vi "XYMovingPart_WangYunong.vi"() -> ()   [LabVIEW 2013]
uses:
  <vilib>/Instr/_visa.llb/VISA Configure Serial Port (Instr).vi
panel:
  in  "Mov speed(mm/s)":dbl format="%#_13g"
  in  "Y pole":refnum<visa-resource-name>
  in  "X pole":refnum<visa-resource-name>
  out "XY Graph":cluster{dbl[], dbl[]}(graph)
  out "Time":dbl
  out "y step":dbl
  out "x step":dbl
  out "Case":i16
  out "Y":i32
  out "X":i32
  out "Chosen Point":dbl[][](array[numeric])
  in  "Size input solution":enum16{"Dynamic Size", "Fixed Size"}(ring)=enum."Fixed Size"
  in  "Polygon Point":dbl[][](array[numeric])
  in  "Y move Maximum / mm":dbl
  in  "X move Maximum / mm":dbl
  in  "Y step / mm":dbl
  in  "X step / mm":dbl
  in  "Initial YPos / mm":dbl
  in  "Initial XPos / mm":dbl
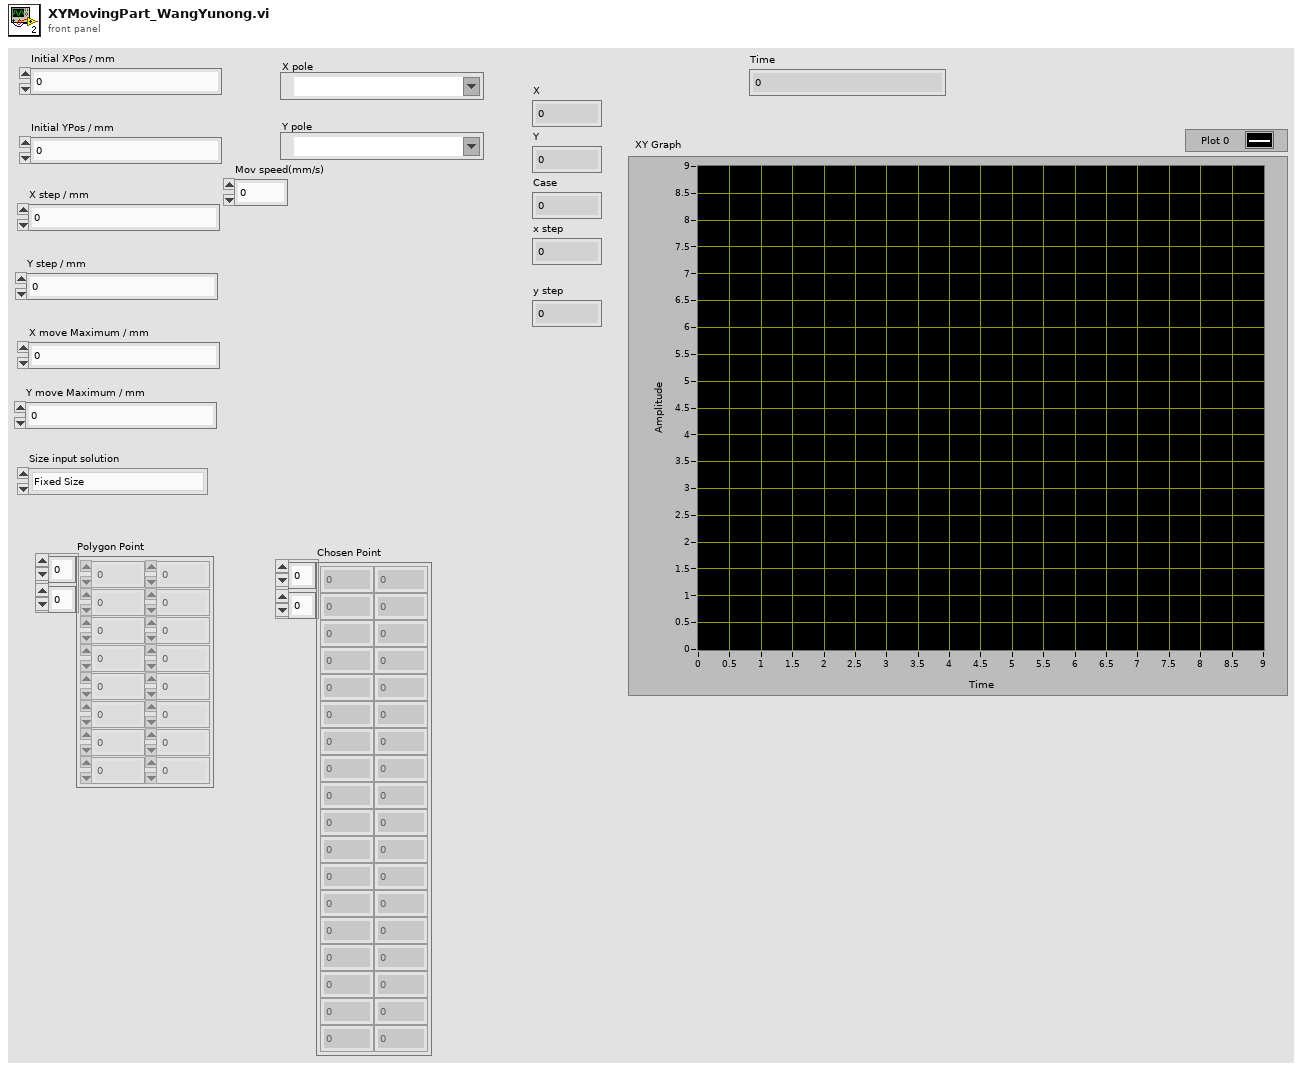
[diagram p1: front panel]
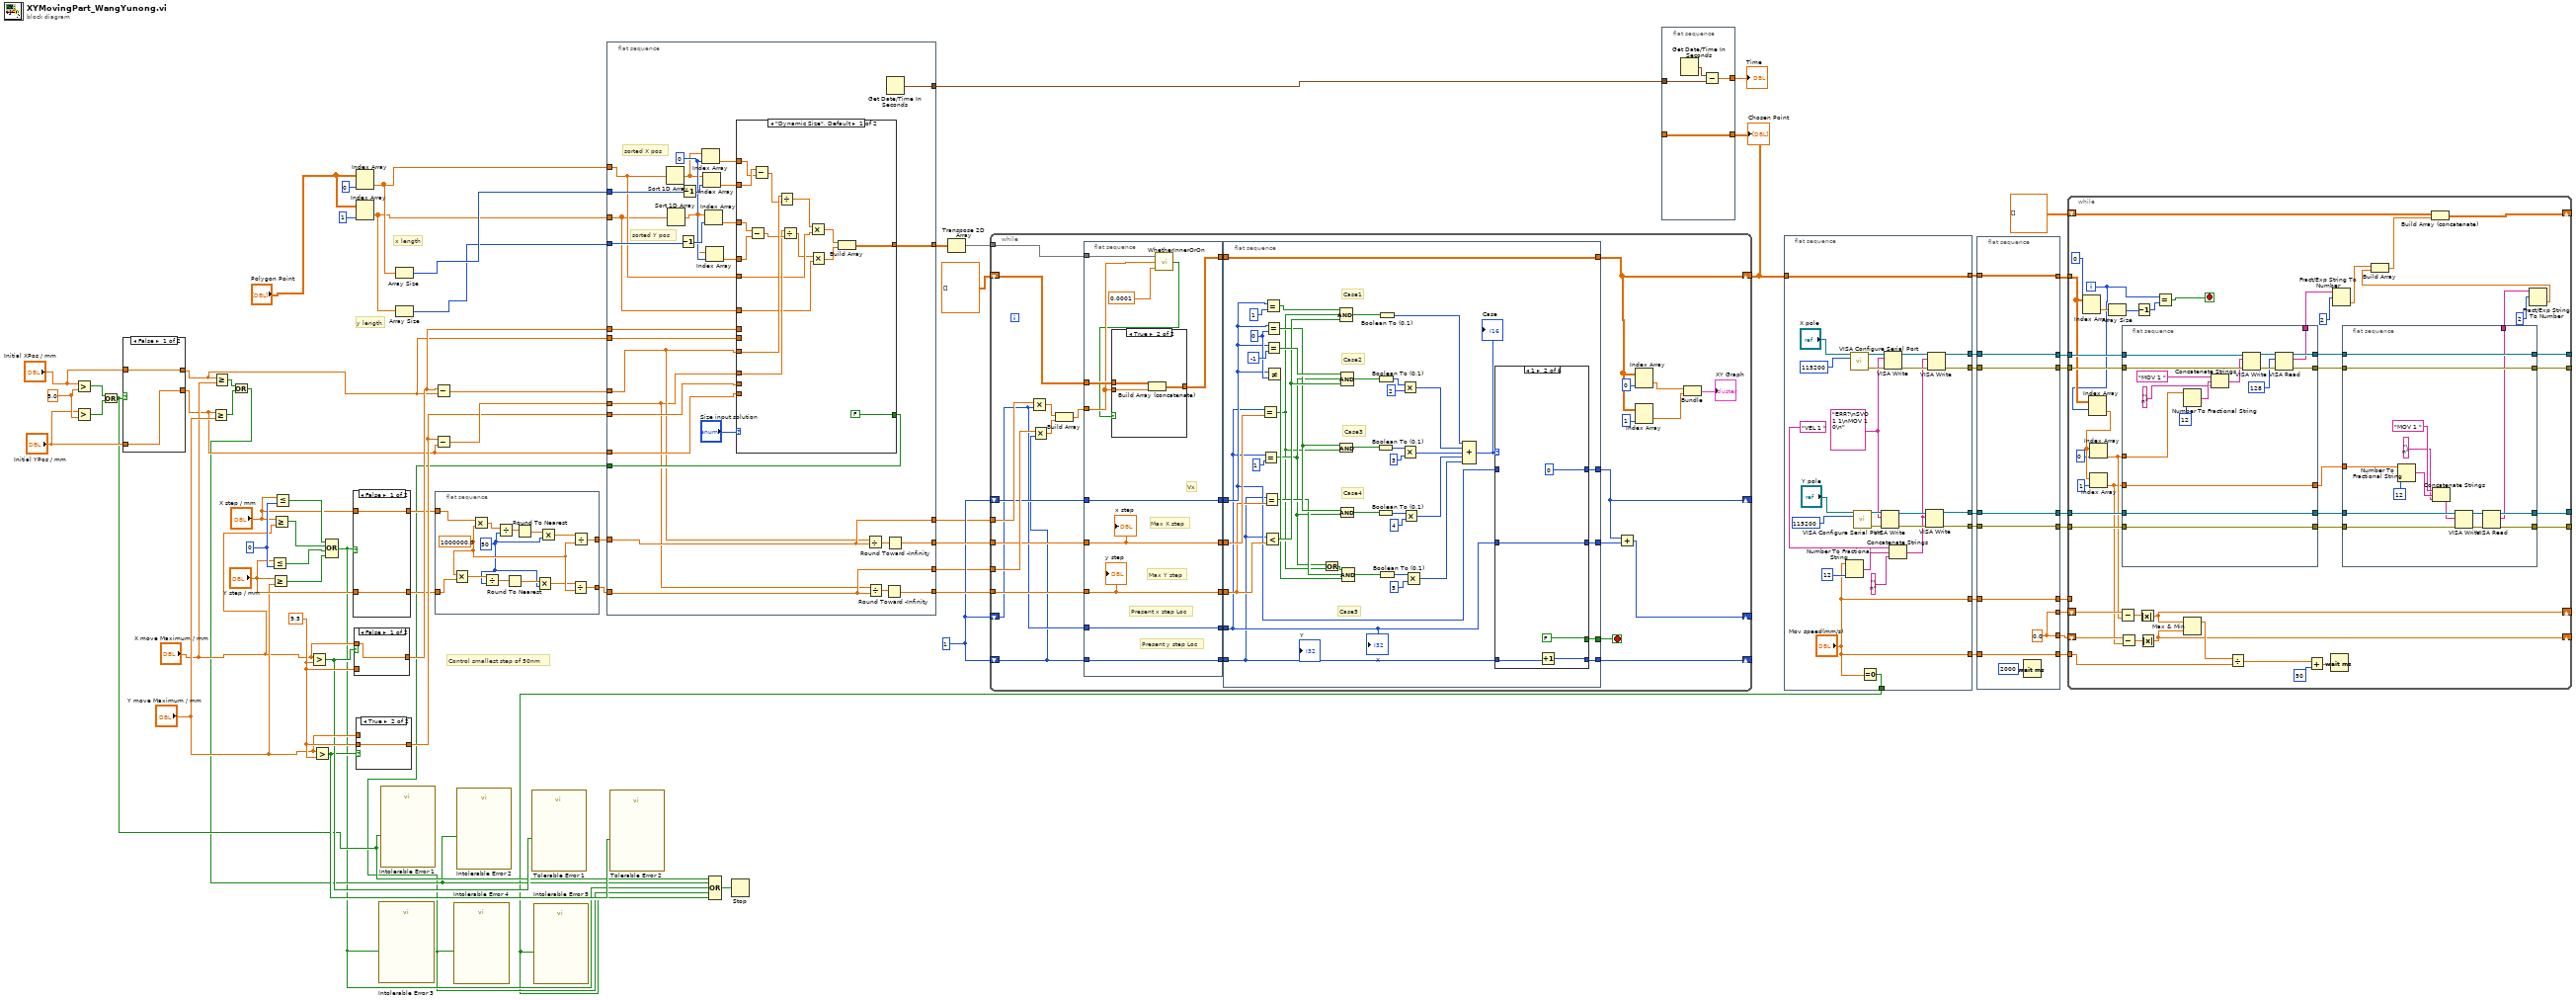
[diagram p0: block diagram]
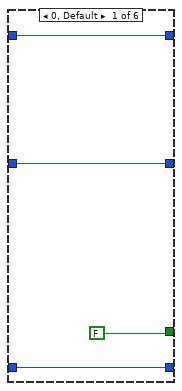
[diagram p2: hidden frame]
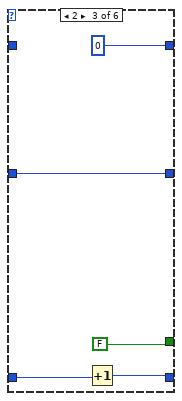
[diagram p3: hidden frame]
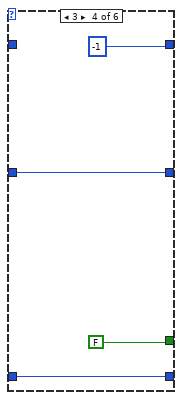
[diagram p4: hidden frame]
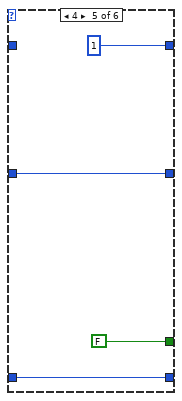
[diagram p5: hidden frame]
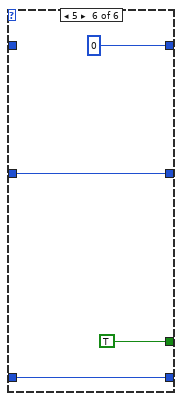
[diagram p6: hidden frame]
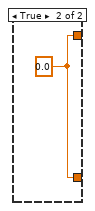
[diagram p8: hidden frame]
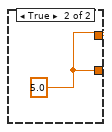
[diagram p11: hidden frame]
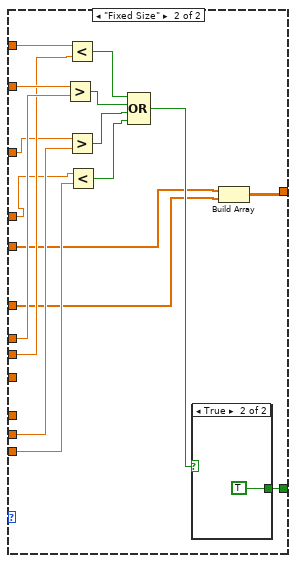
[diagram p12: hidden frame]
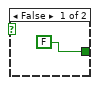
[diagram p13: hidden frame]
diagram:
  w33 = 1
  w65 = 0
  w66 = 9.5
  w71 = 5.0
  # "Control smallest step of 50nm"
  # "y length"
  # "x length"
  n1 = Greater?(x="Initial XPos / mm", y=w71) -> (0:w70:bool)
  n2 = Greater?(x="Initial YPos / mm", y=w71) -> (0:w69:bool)
  n3 = Or(x=w70, y=w69) -> (x .or. y?=w8:bool)
  n4 = case shown="False" w8 {
    tunnel: "Initial XPos / mm" -> [w73 _]
    tunnel: "Initial YPos / mm" -> [w72 _]
    tunnel: [w73 w74] -> w42
    tunnel: [w72 w74] -> w40
    frame False {
    }
    frame True {
      w74 = 5.0
    }
  }
  n5 = Greater Or Equal?(x=w40, y="Y move Maximum / mm") -> (x >= y?=w48:bool)
  n6 = Greater Or Equal?(x=w42, y="X move Maximum / mm") -> (x >= y?=w49:bool)
  n7 = Or(x=w49, y=w48) -> (x .or. y?=w7:bool)
  n8 = Less Or Equal?(x="Y step / mm", y=w65) -> (x <= y?=w62:bool)
  n9 = Greater Or Equal?(x="Y step / mm", y="Y move Maximum / mm") -> (x >= y?=w61:bool)
  n10 = Greater Or Equal?(x="X step / mm", y="X move Maximum / mm") -> (x >= y?=w63:bool)
  n11 = Less Or Equal?(x="X step / mm", y=w65) -> (x <= y?=w64:bool)
  n12 = Greater?(x="X move Maximum / mm", y=w66) -> (0:w45:bool)
  n13 = Greater?(x="Y move Maximum / mm", y=w66) -> (0:w44:bool)
  n14 = Compound Arithmetic op=OR(w64, w63, w62, w61) -> (w6:bool)
  n15 = case shown="False" w6 {
    tunnel: "X step / mm" -> [w76 _]
    tunnel: "Y step / mm" -> [w75 _]
    tunnel: [w76 w77] -> w39
    tunnel: [w75 w77] -> w38
    frame False {
    }
    frame True {
      w77 = 0.0
    }
  }
  n16 = case shown="False" w45 {
    tunnel: w66 -> [_ w79]
    tunnel: "X move Maximum / mm" -> [w78 _]
    tunnel: [w78 w79] -> w43
    frame False {
    }
    frame True {
    }
  }
  n17 = Index Array(array="Polygon Point", index (col)=1 ("disabled index (col)")) -> (element=w54:dbl[])  [unwired: 1 in]
  n18 = case shown="True" w44 {
    tunnel: w66 -> [_ w81]
    tunnel: "Y move Maximum / mm" -> [w80 _]
    tunnel: [w80 w81] -> w41
    frame False {
    }
    frame True {
    }
  }
  n19 = Index Array(array="Polygon Point", index (col)=0 ("disabled index (col)")) -> (element=w56:dbl[])  [unwired: 1 in]
  n20 = call "Intolerable Error 3"("Enable"=w6) -> ()  [unwired: 9 in, 2 out]
  n21 = call "Intolerable Error 1"("Enable"=w8) -> ()  [unwired: 9 in, 2 out]
  n22 = Array Size(array=w56) -> (size(s)=w55:i32)
  n23 = Array Size(array=w54) -> (size(s)=w53:i32)
  n24 = Subtract(x=w43, y=w42) -> (x-y=w47:dbl)
  n25 = Subtract(x=w41, y=w40) -> (x-y=w46:dbl)
  n26 = flat-sequence {
    tunnel: w39 -> [w95]
    tunnel: w38 -> [w92]
    tunnel: [w88] -> w37
    tunnel: [w87] -> w36
    frame #0 {
      w84 = 50
      w89 = 1000000.0
      n27 = Multiply(x=w89, y=w92) -> (x*y=w91:dbl)
      n28 = Multiply(x=w95, y=w89) -> (x*y=w94:dbl)
      n29 = Divide(x=w91, y=w84) -> (x/y=w90:dbl)
      n30 = Divide(x=w94, y=w84) -> (x/y=w93:dbl)
      n31 = Round To Nearest(number=w90) -> (nearest integer value=w85:dbl)
      n32 = Round To Nearest(number=w93) -> (nearest integer value=w86:dbl)
      n33 = Multiply(x=w85, y=w84) -> (x*y=w83:dbl)
      n34 = Multiply(x=w86, y=w84) -> (x*y=w82:dbl)
      n35 = Divide(x=w83, y=w89) -> (x/y=w87:dbl)
      n36 = Divide(x=w82, y=w89) -> (x/y=w88:dbl)
    }
  }
  n37 = call "Intolerable Error 4"("Enable"=w5) -> ()  [unwired: 9 in, 2 out]
  n38 = call "Intolerable Error 2"("Enable"=w7) -> ()  [unwired: 9 in, 2 out]
  n39 = call "Tolerable Error 1"("Enable"=w45) -> ()  [unwired: 9 in, 2 out]
  n40 = call "Intolerable Error 5"("Enable"=w4) -> ()  [unwired: 9 in, 2 out]
  n41 = flat-sequence {
    tunnel: w55 -> [w123]
    tunnel: w53 -> [w121]
    tunnel: w56 -> [w116]
    tunnel: w54 -> [w115]
    tunnel: w47 -> [w99]
    tunnel: w46 -> [w97]
    tunnel: w43 -> [w110]
    tunnel: w42 -> [w109]
    tunnel: w41 -> [w108]
    tunnel: w40 -> [w107]
    tunnel: [w106] -> w5
    tunnel: w37 -> [w100]
    tunnel: w36 -> [w98]
    tunnel: [w105] -> w29
    tunnel: [w102] -> w35
    tunnel: [w101] -> w34
    tunnel: [w98] -> w32
    tunnel: [w100] -> w31
    tunnel: [w96] -> w27
    frame #0 {
      w119 = 0 ("index")
      # "sorted Y pos"
      # "sorted X pos"
      n42 = Sort 1D Array(array=w116) -> (sorted array=w117:dbl[])
      n43 = Sort 1D Array(array=w115) -> (sorted array=w118:dbl[])
      n44 = Decrement(x=w121) -> (x-1=w122:i32)
      n45 = Decrement(x=w123) -> (x-1=w124:i32)
      n46 = Index Array(array=w117, index=w119) -> (element=w113:dbl)
      n47 = Index Array(array=w117, index=w124) -> (element=w114:dbl)
      n48 = Index Array(array=w118, index=w122) -> (element=w112:dbl)
      n49 = Index Array(array=w118, index=w119) -> (element=w111:dbl)
      n50 = case shown="\"Dynamic Size\", Default" "Size input solution" {
        tunnel: w116 -> [w132 w142]
        tunnel: w115 -> [w129 w141]
        tunnel: w114 -> [w140 w157]
        tunnel: w113 -> [w139 w155]
        tunnel: w112 -> [w137 w153]
        tunnel: w111 -> [w138 w150]
        tunnel: w99 -> [w136 _]
        tunnel: w97 -> [w133 _]
        tunnel: [w126 w143] -> w105
        tunnel: w110 -> [_ w156]
        tunnel: w109 -> [_ w154]
        tunnel: w108 -> [_ w152]
        tunnel: w107 -> [_ w151]
        tunnel: [FALSE w144] -> w106
        frame "Dynamic Size", Default {
          n51 = Subtract(x=w137, y=w138) -> (x-y=w134:dbl)
          n52 = Subtract(x=w140, y=w139) -> (x-y=w135:dbl)
          n53 = Divide(x=w136, y=w135) -> (x/y=w131:dbl)
          n54 = Divide(x=w133, y=w134) -> (x/y=w130:dbl)
          n55 = Multiply(x=w131, y=w132) -> (x*y=w128:dbl[])
          n56 = Multiply(x=w130, y=w129) -> (x*y=w127:dbl[])
          n57 = Build Array(w128, w127) -> (w126:dbl[][])
        }
        frame "Fixed Size" {
          n58 = Greater?(x=w157, y=w156) -> (0:w148:bool)
          n59 = Less?(x=w155, y=w154) -> (x < y?=w149:bool)
          n60 = Greater?(x=w153, y=w152) -> (0:w147:bool)
          n61 = Less?(x=w150, y=w151) -> (x < y?=w146:bool)
          n62 = Compound Arithmetic op=OR(w149, w148, w147, w146) -> (w145:bool)
          n63 = case shown="True" w145 {
            tunnel: [FALSE TRUE] -> w144
            frame False {
            }
            frame True {
            }
          }
          n64 = Build Array(w142, w141) -> (w143:dbl[][])
        }
      }
      n65 = Divide(x=w99, y=w100) -> (x/y=w104:dbl)
      n66 = Divide(x=w97, y=w98) -> (x/y=w103:dbl)
      n67 = Round Toward -Infinity(1:w103) -> (0:w101:dbl)
      n68 = Get Date/Time In Seconds() -> (seconds since 1Jan1904=w96:timestamp)
      n69 = Round Toward -Infinity(1:w104) -> (0:w102:dbl)
    }
  }
  n70 = call "Tolerable Error 2"("Enable"=w44) -> ()  [unwired: 9 in, 2 out]
  n71 = Compound Arithmetic op=OR(w8, w7, w6, w5, w4) -> (w3:bool)
  n72 = Stop(stop? (T)=w3) -> ()
  n73 = Transpose 2D Array(2D array=w29) -> (transposed array=w28:dbl[][])
  n74 = while {
    tunnel: w35 -> [w177]
    tunnel: w34 -> [w175]
    tunnel: w28 -> [w183]
    tunnel: w32 -> [w187]
    tunnel: w31 -> [w188]
    shift-right: [w168] -> _
    shift-left: w33 -> [w179]
    shift-right: [w167] -> _
    shift-left: w33 -> [w173]
    shift-right: [w166] -> _
    shift-left: w33 -> [w171]
    shift-right: [w160] -> w24
    shift-left: dbl[][] [] -> [w182]
    stop <- w170 stop-if-true
    n75 = Multiply(x=w188, y=w173) -> (x*y=w186:dbl)
    n76 = Multiply(x=w187, y=w171) -> (x*y=w185:dbl)
    n77 = Build Array(w186, w185) -> (w184:dbl[])
    n78 = flat-sequence {
      tunnel: w184 -> [w259]
      tunnel: w183 -> [w260]
      tunnel: w182 -> [w267]
      tunnel: [w266] -> w181
      tunnel: [w265] -> w180
      tunnel: w179 -> [w265]
      tunnel: [w264] -> w178
      tunnel: w177 -> [w264]
      tunnel: [w263] -> w176
      tunnel: w175 -> [w263]
      tunnel: [w262] -> w174
      tunnel: w173 -> [w262]
      tunnel: [w261] -> w172
      tunnel: w171 -> [w261]
      frame #0 {
        # "Max X step"
        # "Max Y step"
        # "Present y step Loc"
        # "Present x step Loc"
        # "Vx"
        n79 = call "WhetherInnerOrOn.vi"("Error permitted"=0.0001, "JudgePoint"=w259, "InputPolygon"=w260) -> ("Point on or inside?"=w257:bool)
        n80 = case shown="True" w257 {
          tunnel: w267 -> [w268 w271]
          tunnel: w259 -> [_ w270]
          tunnel: [w268 w269] -> w266
          frame False {
          }
          frame True {
            n81 = Build Array (concatenate)(w271, w270) -> (w269:dbl[][])
          }
        }
        "x step" <- w264
        "y step" <- w263
      }
    }
    n82 = flat-sequence {
      tunnel: w181 -> [w189]
      tunnel: w180 -> [w196]
      tunnel: w178 -> [w227]
      tunnel: w176 -> [w224]
      tunnel: w174 -> [w195]
      tunnel: w172 -> [w194]
      tunnel: [w193] -> w170
      tunnel: [w192] -> w169
      tunnel: [w191] -> w168
      tunnel: [w190] -> w166
      tunnel: [w189] -> w160
      frame #0 {
        w228 = 0
        # "Case5"
        # "Case4"
        # "Case3"
        # "Case2"
        # "Case1"
        n83 = Equal?(x=w195, y=w227) -> (x = y?=w216:bool)
        n84 = Equal?(x=w195, y=1) -> (x = y?=w217:bool)
        n85 = Equal?(x=w194, y=w224) -> (x = y?=w218:bool)
        n86 = Less?(x=w194, y=w224) -> (x < y?=w222:bool)
        n87 = Equal?(x=w196, y=1) -> (x = y?=w225:bool)
        n88 = Equal?(x=w196, y=w228) -> (x = y?=w221:bool)
        n89 = Equal?(x=w196, y=-1) -> (x = y?=w223:bool)
        n90 = Not Equal?(x=w196, y=w228) -> (x != y?=w219:bool)
        n91 = Or(x=w217, y=w216) -> (x .or. y?=w220:bool)
        n92 = Compound Arithmetic op=AND(w225, w216, w222) -> (w215:bool)
        n93 = Compound Arithmetic op=AND(w221, w216) -> (w213:bool)
        n94 = Compound Arithmetic op=AND(w223, w217, w222) -> (w214:bool)
        n95 = Compound Arithmetic op=AND(w221, w217) -> (w212:bool)
        n96 = Compound Arithmetic op=AND(w220, w218, w219) -> (w211:bool)
        n97 = Boolean To (0,1)(Boolean=w213) -> (0, 1=w206:i16)
        n98 = Boolean To (0,1)(Boolean=w212) -> (0, 1=w204:i16)
        n99 = Boolean To (0,1)(Boolean=w214) -> (0, 1=w208:i16)
        n100 = Boolean To (0,1)(Boolean=w215) -> (0, 1=w209:i16)
        n101 = Boolean To (0,1)(Boolean=w211) -> (0, 1=w202:i16)
        n102 = Multiply(x=w208, y=i16 2) -> (x*y=w200:i16)
        n103 = Multiply(x=w206, y=i16 3) -> (x*y=w199:i16)
        n104 = Multiply(x=w204, y=i16 4) -> (x*y=w198:i16)
        n105 = Multiply(x=w202, y=i16 5) -> (x*y=w197:i16)
        n106 = Compound Arithmetic op=ADD(w209, w200, w199, w198, w197) -> (w210:i16)
        "Case" <- w210
        n107 = case shown="1" w210 {
          tunnel: w196 -> [w234 _ _ _ _ _]
          tunnel: w195 -> [w233 w236 w241 w247 w251 w256]
          tunnel: w194 -> [w232 w238 w243 w246 w250 w255]
          tunnel: [w234 0 0 -1 1 0] -> w191
          tunnel: [w233 w236 w241 w247 w251 w256] -> w192
          tunnel: [w232 w237 w242 w246 w250 w255] -> w190
          tunnel: [FALSE FALSE FALSE FALSE FALSE TRUE] -> w193
          frame 0, Default {
          }
          frame 1 {
            n108 = Increment(x=w238) -> (x+1=w237:i32)
          }
          frame 2 {
            n109 = Increment(x=w243) -> (x+1=w242:i32)
          }
          frame 3 {
          }
          frame 4 {
          }
          frame 5 {
          }
        }
        "X" <- w195
        "Y" <- w194
      }
    }
    n110 = Add(x=w168, y=w169) -> (x+y=w167:i32)
    n111 = Index Array(array=w160, index (col)=0 ("disabled index (col)")) -> (element=w163:dbl[])  [unwired: 1 in]
    n112 = Index Array(array=w160, index (col)=1 ("disabled index (col)")) -> (element=w162:dbl[])  [unwired: 1 in]
    n113 = Bundle(w163, w162) -> (→"XY Graph":cluster{dbl[], dbl[]})  [unwired: 1 in]
  }
  n114 = flat-sequence {
    tunnel: [w275] -> w25
    tunnel: w24 -> [w275]
    tunnel: w27 -> [w273]
    tunnel: [w272] -> w26
    frame #0 {
      n115 = Get Date/Time In Seconds() -> (seconds since 1Jan1904=w274:timestamp)
      n116 = Subtract(x=w274, y=w273) -> (x-y=w272:dbl)
    }
  }
  n117 = flat-sequence {
    tunnel: [w291] -> w23
    tunnel: w24 -> [w291]
    tunnel: [w284] -> w22
    tunnel: [w283] -> w21
    tunnel: [w288] -> w20
    tunnel: [w287] -> w19
    tunnel: ["Mov speed(mm/s)"] -> w12
    tunnel: [w277] -> w4
    tunnel: ["Mov speed(mm/s)"] -> w2
    frame #0 {
      w292 = "ERR?\nSVO 1 1\nMOV 1 0\n"
      n118 = Number To Fractional String(number="Mov speed(mm/s)", precision (6)=i16 12) -> (F-format string=w281:string)  [unwired: 2 in]
      n119 = call-poly "VISA Configure Serial Port"("VISA resource name"="X pole", "baud rate (9600)"=u32 115200) -> ("VISA resource name out"=w296:refnum<visa-resource-name>, "error out"=w295:errorcluster)  [unwired: 12 in]
      n120 = call-poly "VISA Configure Serial Port"("VISA resource name"="Y pole", "baud rate (9600)"=u32 115200) -> ("VISA resource name out"=w294:refnum<visa-resource-name>, "error out"=w293:errorcluster)  [unwired: 12 in]
      n121 = Equal To 0?(x="Mov speed(mm/s)") -> (x = 0?=w277:bool)
      n122 = VISA Write(VISA resource name=w294, write buffer=w292, error in (no error)=w293) -> (VISA resource name out=w290:refnum<visa-resource-name>, error out=w289:errorcluster)  [unwired: 1 out]
      n123 = VISA Write(VISA resource name=w296, write buffer=w292, error in (no error)=w295) -> (VISA resource name out=w286:refnum<visa-resource-name>, error out=w285:errorcluster)  [unwired: 1 out]
      n124 = Concatenate Strings("VEL 1 ", w281, "\n") -> (w278:string)
      n125 = VISA Write(VISA resource name=w290, write buffer=w278, error in (no error)=w289) -> (VISA resource name out=w288:refnum<visa-resource-name>, error out=w287:errorcluster)  [unwired: 1 out]
      n126 = VISA Write(VISA resource name=w286, write buffer=w278, error in (no error)=w285) -> (VISA resource name out=w284:refnum<visa-resource-name>, error out=w283:errorcluster)  [unwired: 1 out]
    }
  }
  n127 = flat-sequence {
    tunnel: [w309] -> w18
    tunnel: w23 -> [w309]
    tunnel: [w308] -> w17
    tunnel: w22 -> [w308]
    tunnel: w21 -> [w307]
    tunnel: [w307] -> w16
    tunnel: w20 -> [w306]
    tunnel: [w306] -> w15
    tunnel: [w305] -> w14
    tunnel: w19 -> [w305]
    tunnel: w12 -> [w303]
    tunnel: [w303] -> w11
    tunnel: [w302] -> w10
    tunnel: [w302] -> w9
    tunnel: w2 -> [w301]
    tunnel: [w301] -> w1
    frame #0 {
      w302 = 0.0
      n128 = Wait (ms)(milliseconds to wait=u32 2000) -> ()  [unwired: 1 out]
    }
  }
  n129 = while {
    tunnel: w18 -> [w345]
    tunnel: w17 -> [w349]
    tunnel: w16 -> [w348]
    tunnel: w15 -> [w347]
    tunnel: w14 -> [w346]
    tunnel: [w339] -> _
    tunnel: [w338] -> _
    tunnel: [w336] -> _
    tunnel: [w334] -> _
    tunnel: w11 -> [_]
    shift-right: [w321] -> _
    shift-left: dbl[][] [] -> [w322]
    tunnel: w1 -> [w313]
    shift-right: [w310] -> _
    shift-left: w10 -> [w320]
    shift-right: [w311] -> _
    shift-left: w9 -> [w319]
    i -> [w344]
    stop <- w350 stop-if-true
    n130 = Index Array(array=w345, index (col)=0 ("disabled index (col)")) -> (element=w353:dbl[])  [unwired: 1 in]
    n131 = Index Array(array=w345, index (row)=w344) -> (element=w330:dbl[])  [unwired: 1 in]
    n132 = Index Array(array=w330, index=0) -> (element=w318:dbl)
    n133 = Index Array(array=w330, index=1) -> (element=w317:dbl)
    n134 = Array Size(array=w353) -> (size(s)=w352:i32)
    n135 = Subtract(x=w320, y=w318) -> (x-y=w316:dbl)
    n136 = Subtract(x=w319, y=w317) -> (x-y=w315:dbl)
    n137 = flat-sequence {
      tunnel: w349 -> [w386]
      tunnel: w348 -> [w385]
      tunnel: w347 -> [w373]
      tunnel: w346 -> [w372]
      tunnel: [w377] -> w343
      tunnel: [w376] -> w342
      tunnel: [w375] -> w341
      tunnel: [w373] -> w335
      tunnel: [w372] -> w337
      tunnel: w318 -> [w371]
      tunnel: [w370] -> w328
      tunnel: w317 -> [w370]
      frame #0 {
        n138 = Number To Fractional String(number=w371, precision (6)=i16 12) -> (F-format string=w382:string)  [unwired: 2 in]
        n139 = Concatenate Strings("MOV 1 ", w382, "\n") -> (w384:string)
        n140 = VISA Write(VISA resource name=w386, write buffer=w384, error in (no error)=w385) -> (VISA resource name out=w379:refnum<visa-resource-name>, error out=w380:errorcluster)  [unwired: 1 out]
        n141 = VISA Read(VISA resource name=w379, byte count=u32 128, error in (no error)=w380) -> (VISA resource name out=w377:refnum<visa-resource-name>, read buffer=w375:string, error out=w376:errorcluster)  [unwired: 1 out]
      }
    }
    n142 = Decrement(x=w352) -> (x-1=w351:i32)
    n143 = Absolute Value(x=w316) -> (abs(x)=w310:dbl)
    n144 = Absolute Value(x=w315) -> (abs(x)=w311:dbl)
    n145 = Equal?(x=w344, y=w351) -> (x = y?=w350:bool)
    n146 = Max & Min(x=w310, y=w311) -> (max(x,y)=w314:dbl)  [unwired: 1 out]
    n147 = Divide(x=w314, y=w313) -> (x/y=w312:dbl)
    n148 = Add(x=w312, y=50) -> (x+y=w333:dbl)
    n149 = Wait (ms)(milliseconds to wait=w333) -> ()  [unwired: 1 out]
    n150 = Fract/Exp String To Number(string=w341, offset=2) -> (number=w324:dbl)  [unwired: 2 in, 1 out]
    n151 = flat-sequence {
      tunnel: w343 -> [w368]
      tunnel: w342 -> [w367]
      tunnel: [w368] -> w339
      tunnel: [w367] -> w338
      tunnel: w337 -> [w362]
      tunnel: [w359] -> w336
      tunnel: w335 -> [w363]
      tunnel: [w358] -> w334
      tunnel: w328 -> [w356]
      tunnel: [w355] -> w326
      frame #0 {
        n152 = Number To Fractional String(number=w356, precision (6)=i16 12) -> (F-format string=w366:string)  [unwired: 2 in]
        n153 = Concatenate Strings("MOV 1 ", w366, "\n" ("string")) -> (w357:string)
        n154 = VISA Write(VISA resource name=w363, write buffer=w357, error in (no error)=w362) -> (VISA resource name out=w361:refnum<visa-resource-name>, error out=w360:errorcluster)  [unwired: 1 out]
        n155 = VISA Read(VISA resource name=w361, error in (no error)=w360) -> (VISA resource name out=w359:refnum<visa-resource-name>, read buffer=w355:string, error out=w358:errorcluster)  [unwired: 1 in, 1 out]
      }
    }
    n156 = Fract/Exp String To Number(string=w326, offset=2) -> (number=w325:dbl)  [unwired: 2 in, 1 out]
    n157 = Build Array(w324, w325) -> (w323:dbl[])
    n158 = Build Array (concatenate)(w322, w323) -> (w321:dbl[][])
  }
  "Chosen Point" <- w25
  "Time" <- w26
